vi "Write Gral. (SubVI).vi"(8 "error in (no error)":errorcluster, 10 "Combo Box":string(combo)="S", 11 "VISA Refnum in":refnum<visa-resource-name>) -> (0 "error out":errorcluster, 3 "VISA Refnum out":refnum<visa-resource-name>)   [LabVIEW 2014]
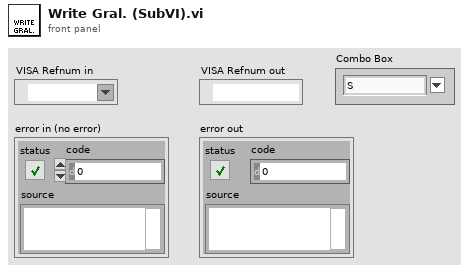
[diagram p1: front panel]
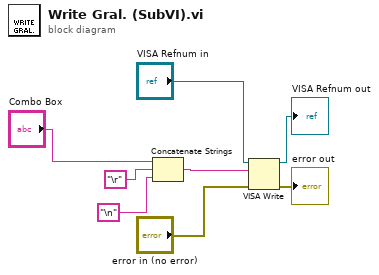
[diagram p0: block diagram]
diagram:
  n1 = Concatenate Strings("Combo Box", "\r", "\n") -> (w3:string)
  n2 = VISA Write(VISA resource name="VISA Refnum in", write buffer=w3, error in (no error)="error in (no error)") -> (VISA resource name out=→"VISA Refnum out":refnum<visa-resource-name>, error out=→"error out":errorcluster)  [unwired: 1 out]
